vi "高速数据通信 外部批处理.vi"() -> ()   [LabVIEW 2016]
doc: "This example mainly indicates how to acquire profiles from controllers by using <B>Read Profiles (for High-Speed Communication)</B> VI via high-speed communication."
uses:
  Public/Clusters/Ethernet Config.ctl
  Public/Clusters/High-Speed Comm Start Req.ctl
  Public/Constants/High-Speed Comm Start Pos.ctl
  Public/Constants/High-Speed Receive Ratio.ctl
  Public/Clusters/Profile Info.ctl
  KEYENCE LJ-X8000A.lvlib
panel:
  out "Luminance Image":u16[][](graph)
  out "error out":errorcluster
  out "Comm":bool
  out "Monitoring":bool
  out "Timeout Cnt":u32
  out "Height Image":dbl[][](graph)
  out "Read Cnt":u32
  out "Notify":u32
  out "Buf Usage Rate":u32
  out "Profile Info":T1
  in  "Start Req":T2={"High-Speed Comm Start Pos"=2, "Read Profile Cnt"=1000, "High-Speed Receive Ratio"=16} {"High-Speed Receive Ratio" items=["LOWEST"=0, "LOW"=16, "MIDDLE"=17, "HIGH"=18, "HIGHEST"=32]; "High-Speed Comm Start Pos" items=["SEND COMPLETE POS", "OLDEST", "NEXT"]}
  in  "Port No":u16=24692
  in  "Stop Monitoring":bool
  in  "Start Monitoring":bool
  in  "Stop High Speed Comm":bool
  in  "Start High Speed Comm":bool
  in  "Stop VI":bool
  in  "Ethernet Config":T5={"IP Address"=[192, 168, 0, 1], "Port No"=24691}
  # "Read Profiles Start/Stop"
  # "High Speed Data Communication Start/Stop"
  # "Communication Configuration"
  # "Output from Read Profiles VI"
  # "Communication Configuration\nfor High Speed Communication"
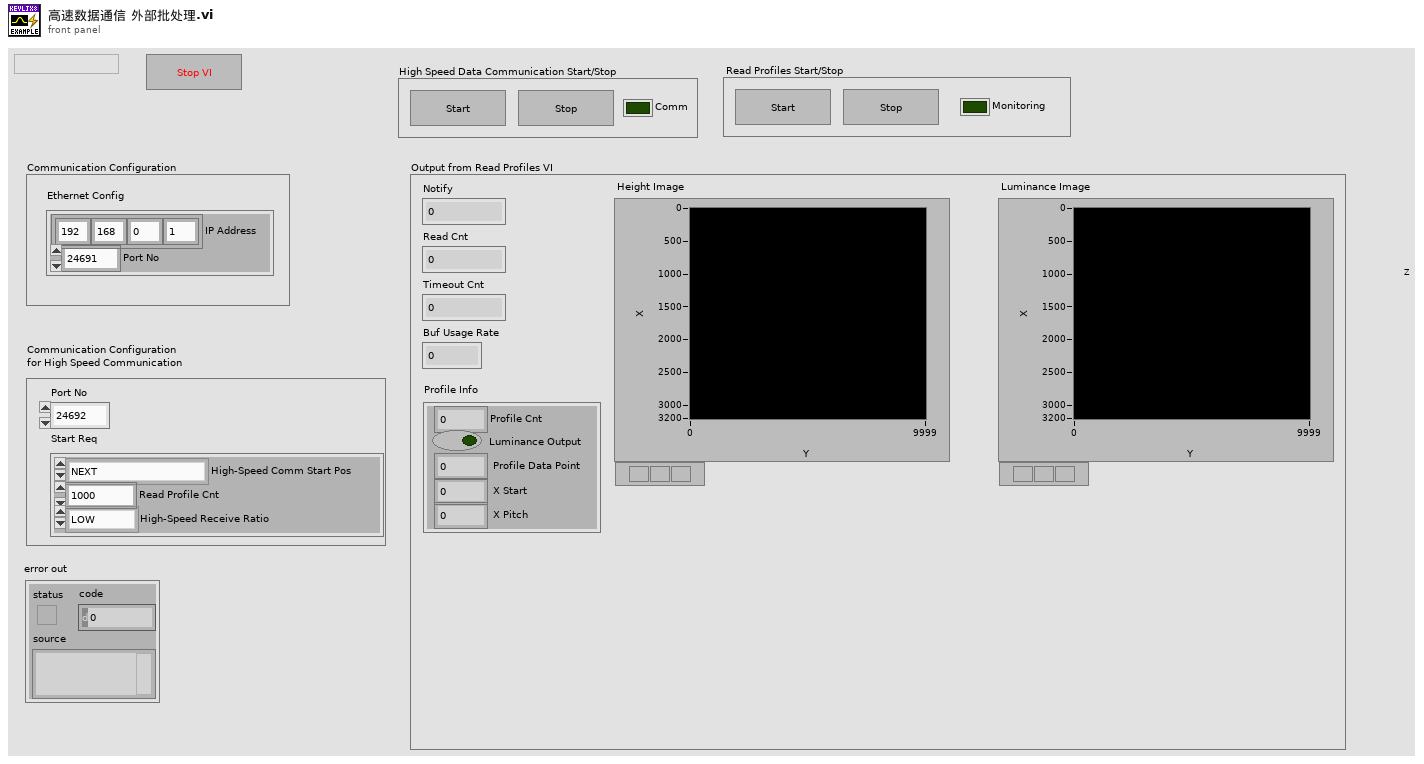
[diagram p1: front panel]
types:
  T1 = typedef "KEYENCE LJ-X8000A.lvlib/Profile Info.ctl" = cluster{"Profile Cnt":u8, "Luminance Output":bool, " Profile Data Point":u16, " X Start":i32, " X Pitch":i32}
  T2 = typedef "KEYENCE LJ-X8000A.lvlib/High-Speed Comm Start Req.ctl" = cluster{"High-Speed Comm Start Pos":T3, "Read Profile Cnt":u32, "High-Speed Receive Ratio":T4}
  T3 = typedef "KEYENCE LJ-X8000A.lvlib/High-Speed Comm Start Pos.ctl" = u8
  T4 = typedef "KEYENCE LJ-X8000A.lvlib/High-Speed Receive Ratio.ctl" = u8
  T5 = typedef "KEYENCE LJ-X8000A.lvlib/Ethernet Config.ctl" = cluster{"IP Address":u8[], "Port No":u16}
  T6 = enum8{"Enabled", "Disabled", "Disabled and Grayed Out"}
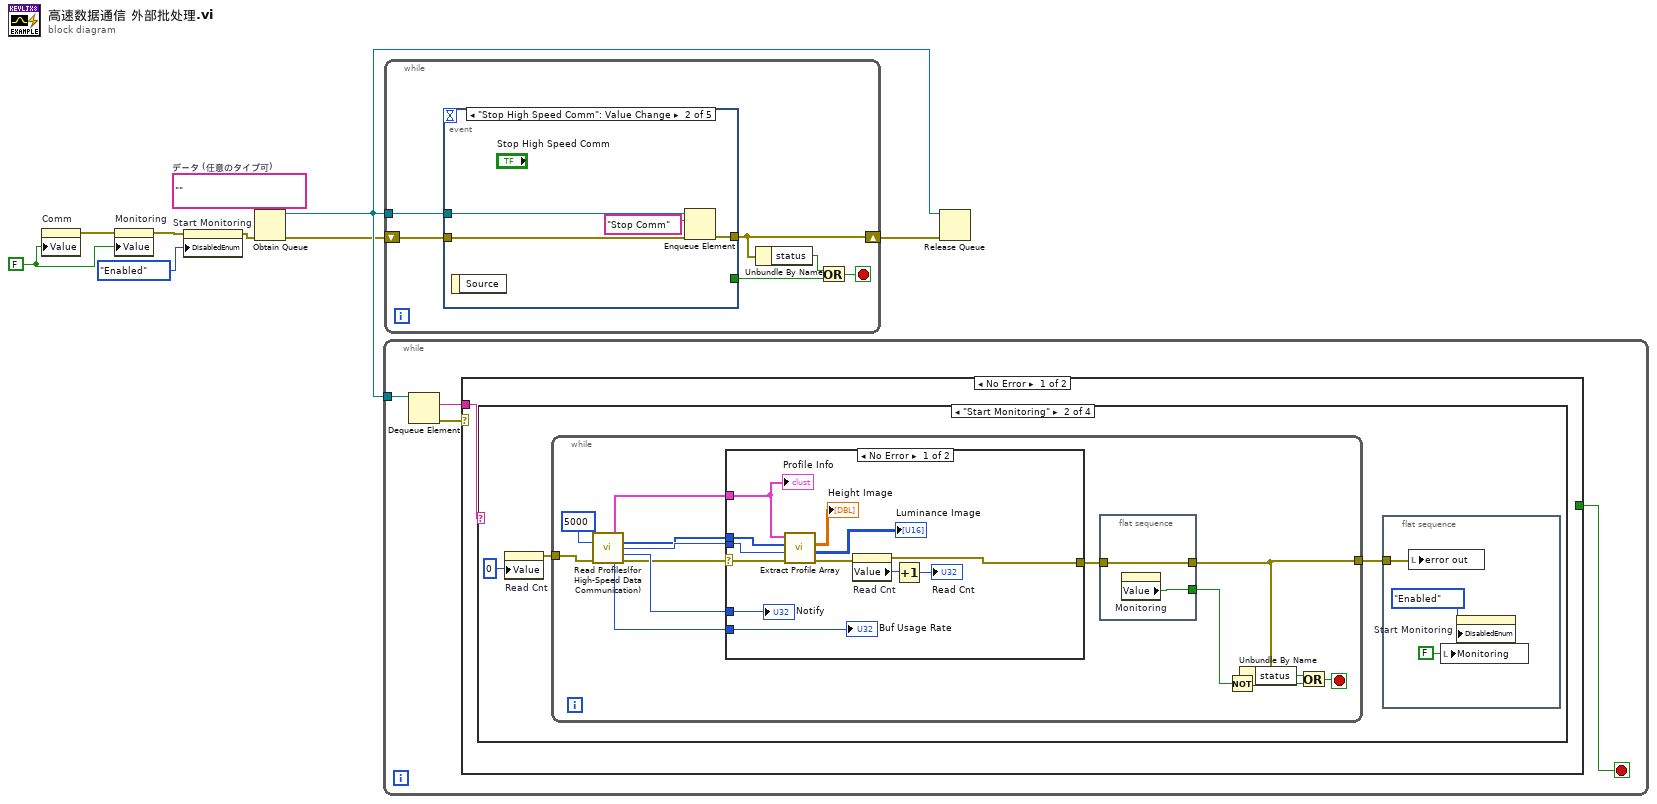
[diagram p0: block diagram]
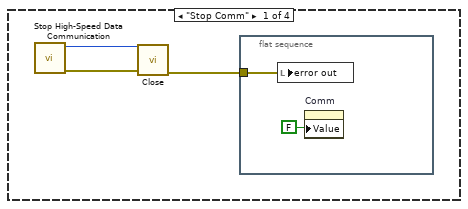
[diagram p2: hidden frame]
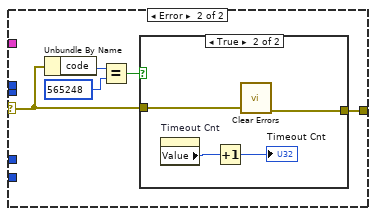
[diagram p3: hidden frame]
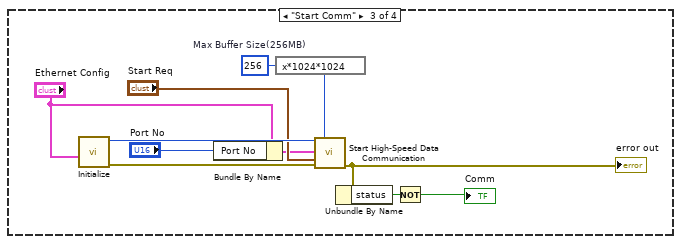
[diagram p5: hidden frame]
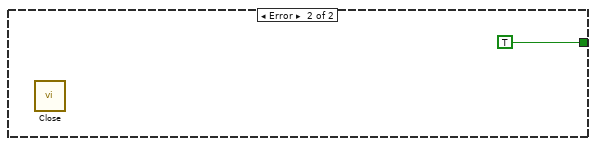
[diagram p7: hidden frame]
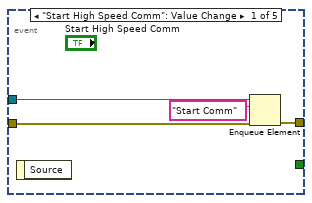
[diagram p8: hidden frame]
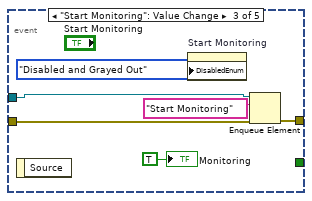
[diagram p9: hidden frame]
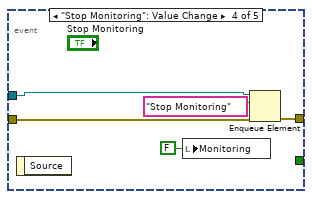
[diagram p10: hidden frame]
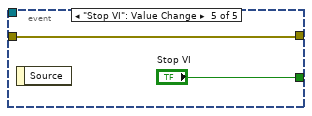
[diagram p11: hidden frame]
diagram:
  w5 = FALSE ("Monitoring")
  w7 = ""  # データ (任意のタイプ可)
  n1 = property on="Comm" class="Bool (strict)"("Value"=w5) -> (error out=w6:errorcluster)  [unwired: 2 in, 1 out]
  n2 = property on="Monitoring" class="Bool (strict)"(error in=w6, "Value"=w5) -> (error out=w4:errorcluster)  [unwired: 1 in, 1 out]
  n3 = property on="Start Monitoring" class="Bool"(error in=w4, "DisabledEnum"=T6."Enabled" ("–³Œø")) -> (error out=w2:errorcluster)  [unwired: 1 in, 1 out]
  n4 = Obtain Queue(element data type=w7, error in (no error)=w2) -> (queue out=w8:refnum<queue>, error out=w3:errorcluster)  [unwired: 3 in, 1 out]
  n5 = while {
    tunnel: w8 -> [w13]
    stop <- w10 stop-if-true
    n6 = Dequeue Element(queue=w13) -> (element=w11:string, error out=w12:errorcluster)  [unwired: 2 in, 2 out]
    n7 = case shown="No Error" w12 {
      tunnel: w11 -> [w14 _]
      tunnel: [_ TRUE] -> w10
      frame No Error {
        n8 = case shown="\"Start Monitoring\"" w14 {
          frame "Stop Comm" {
            n9 = call "Stop High-Speed Data Communication.vi"() -> ("error out"=w17:errorcluster, "Device ID out"=w16:i32)  [unwired: 10 in]
            n10 = call "Close.vi"("error in (no error)"=w17, "Device ID (0)"=w16) -> ("error out"=w15:errorcluster)  [unwired: 8 in, 1 out]
            n11 = flat-sequence {
              tunnel: w15 -> [w19]
              frame #0 {
                n12 = local write "error out"(w19) -> ()
                n13 = property on="Comm" class="Bool (strict)"("Value"=FALSE ("Comm")) -> ()  [unwired: 2 in, 2 out]
              }
            }
          }
          frame "Start Monitoring" {
            n14 = property on="Read Cnt" class="DigNum (strict)"("Value"=u32 0 ("Read Cnt")) -> (error out=w21:errorcluster)  [unwired: 2 in, 1 out]
            n15 = while {
              tunnel: w21 -> [w34]
              tunnel: [w29] -> w22
              stop <- w31 stop-if-true
              n16 = call "Read Profiles(for High-Speed Data Communication).vi"("Timeout"=u32 5000, "error in (no error)"=w34) -> ("Profile Info"=w38:T1, "Profile Data"=w32:u32[], "Rsp Profile Cnt"=w35:u32, "Notify"=w36:u32, "Buf Usage Rate"=w39:u32, "error out"=w27:errorcluster)  [unwired: 7 in, 1 out]
              n17 = case shown="No Error" w27 {
                selector: w27 -> [w48 w58]
                tunnel: w39 -> [w53 _]
                tunnel: w38 -> [w47 _]
                tunnel: w36 -> [w52 _]
                tunnel: w35 -> [w45 _]
                tunnel: [w49 w57] -> w30
                tunnel: w32 -> [w46 _]
                frame No Error {
                  n18 = call "Extract Profile Array.vi"("error in (no error)"=w48, "Profile Cnt"=w45, "Profile Data"=w46, "Profile Info"=w47) -> ("error out"=w44:errorcluster, "Luminance Profile Array"=→"Luminance Image":u16[][], "Height Profile Array"=→"Height Image":dbl[][])  [unwired: 4 in, 1 out]
                  n19 = property on="Read Cnt" class="DigNum (strict)"(error in=w44) -> (error out=w49:errorcluster, "Value"=w51:u32)  [unwired: 1 in, 1 out]
                  n20 = Increment(x=w51) -> (x+1=→"Read Cnt":u32)
                  "Buf Usage Rate" <- w53
                  "Profile Info" <- w47
                  "Notify" <- w52
                }
                frame Error {
                  n21 = Unbundle By Name(w58) -> ("code"=w56:i32)
                  n22 = Equal?(x=w56, y=565248) -> (x = y?=w54:bool)
                  n23 = case shown="True" w54 {
                    tunnel: w58 -> [w59 w63]
                    tunnel: [w59 w62] -> w57
                    frame False {
                    }
                    frame True {
                      n24 = property on="Timeout Cnt" class="DigNum (strict)"() -> ("Value"=w61:u32)  [unwired: 2 in, 2 out]
                      n25 = Increment(x=w61) -> (x+1=→"Timeout Cnt":u32)
                      n26 = call <vilib>:"Clear Errors.vi"("error in (no error)"=w63) -> ("error out"=w62:errorcluster)  [unwired: 5 in, 1 out]
                    }
                  }
                }
              }
              n27 = flat-sequence {
                tunnel: w30 -> [w41]
                tunnel: [w41] -> w29
                tunnel: [w40] -> w28
                frame #0 {
                  n28 = property on="Monitoring" class="Bool (strict)"() -> ("Value"=w40:bool)  [unwired: 2 in, 2 out]
                }
              }
              n29 = Not(x=w28) -> (.not. x?=w33:bool)
              n30 = Unbundle By Name(w29) -> ("status"=w26:bool)
              n31 = Or(x=w26, y=w33) -> (x .or. y?=w31:bool)
            }
            n32 = flat-sequence {
              tunnel: w22 -> [w23]
              frame #0 {
                n33 = local write "error out"(w23) -> ()
                n34 = local write "Monitoring"(FALSE ("Monitoring")) -> ()
                n35 = property on="Start Monitoring" class="Bool"("DisabledEnum"=T6."Enabled" ("–³Œø")) -> ()  [unwired: 2 in, 2 out]
              }
            }
          }
          frame "Start Comm" {
            w65 = u32 256  # Max Buffer Size(256MB)
            n36 = call "Initialize.vi"("Ethernet Config"="Ethernet Config") -> ("error out"=w67:errorcluster, "Device ID out"=w74:i32)  [unwired: 9 in]
            n37 = Bundle By Name(cluster="Ethernet Config", "Port No"="Port No") -> (w70:T5)
            n38 = expression code="x*1024*1024"(w65) -> (w69:u32)
            n39 = call "Start High-Speed Data Communication.vi"("Device ID"=w74, "Max Buffer Size"=w69, "Ethernet Config"=w70, "Start Req"="Start Req", "error in (no error)"=w67) -> ("error out"=w66:errorcluster)  [unwired: 9 in, 1 out]
            "error out" <- w66
            n40 = Unbundle By Name(w66) -> ("status"=w64:bool)
            n41 = Not(x=w64) -> (.not. x?=→"Comm":bool)
          }
          frame Default {
          }
        }
      }
      frame Error {
        n42 = call "Close.vi"() -> ()  [unwired: 10 in, 2 out]
      }
    }
  }
  n43 = while {
    shift-right: [w77] -> w9
    shift-left: w3 -> [w80]
    tunnel: w8 -> [w81]
    stop <- w78 stop-if-true
    n44 = event shown="[1] \"Stop High Speed Comm\": Value Change" {
      selector: _ -> [_ _ _ _ _]
      dyn-events: _ -> [_ _ _ _ _]
      timeout: _ -> [_ _ _ _ _]
      tunnel: w81 -> [w85 w89 w91 w96 _]
      tunnel: w80 -> [w84 w88 w95 w100 w102]
      tunnel: [w83 w87 w94 w99 w102] -> w77
      tunnel: [_ _ _ _ "Stop VI"] -> w79
      event "Start High Speed Comm": Value Change {
        n45 = event-data() -> ()  [unwired: 1 in, 1 out]
        n46 = Enqueue Element(queue=w85, element="Start Comm", error in (no error)=w84) -> (error out=w83:errorcluster)  [unwired: 1 in, 2 out]
      }
      event "Stop High Speed Comm": Value Change {
        n47 = event-data() -> ()  [unwired: 1 in, 1 out]
        n48 = Enqueue Element(queue=w89, element="Stop Comm", error in (no error)=w88) -> (error out=w87:errorcluster)  [unwired: 1 in, 2 out]
      }
      event "Start Monitoring": Value Change {
        n49 = event-data() -> ()  [unwired: 1 in, 1 out]
        n50 = property on="Start Monitoring" class="Bool"("DisabledEnum"=T6."Disabled and Grayed Out" ("–³Œø")) -> ()  [unwired: 2 in, 2 out]
        n51 = Enqueue Element(queue=w91, element="Start Monitoring", error in (no error)=w95) -> (error out=w94:errorcluster)  [unwired: 1 in, 2 out]
        "Monitoring" <- TRUE ("Monitoring")
      }
      event "Stop Monitoring": Value Change {
        n52 = event-data() -> ()  [unwired: 1 in, 1 out]
        n53 = local write "Monitoring"(FALSE ("Monitoring")) -> ()
        n54 = Enqueue Element(queue=w96, element="Stop Monitoring", error in (no error)=w100) -> (error out=w99:errorcluster)  [unwired: 1 in, 2 out]
      }
      event "Stop VI": Value Change {
        n55 = event-data() -> ()  [unwired: 1 in, 1 out]
      }
    }
    n56 = Unbundle By Name(w77) -> ("status"=w76:bool)
    n57 = Or(x=w76, y=w79) -> (x .or. y?=w78:bool)
  }
  n58 = Release Queue(queue=w8, error in (no error)=w9) -> ()  [unwired: 1 in, 3 out]
